vi "cXB_trt-2-dist.vi"(8 "err in":errorcluster, 11 "cXB (e)":T1) -> (0 "errout":errorcluster caption="err out", 3 "cXB (s)":T1)   [LabVIEW 2010]
doc: "Calcul des caractéristiques de la distribution expérimentale : nic (effectifs cumulés), Densité de probabilité f(X), Fonction de répartition F(X) à partir des informations en entrée (n obs. ou nc classes), de l'effectif total (n), et du tableau 1D des effectifs associés (ni) à chaque valeur ou chaque classe."
uses:
  lv_04/commandes/cX.ctl
  lv_04/commandes/cSTA_varid.ctl
  lv_04/commandes/c_TDMS_ch_variable.ctl
  lv_04/commandes/c_TDMS_ch_donnees.ctl
  lv_04/commandes/c0-var-n.ctl
  lv_04/commandes/cSTA_num_do_cr.ctl
  lv_04/commandes/c02-do-num.ctl
  lv_04/commandes/c04-stat-num.ctl
  lv_04/commandes/cSTA_txt_do_cr.ctl
  lv_04/commandes/c02-do-txt.ctl
  lv_04/commandes/c04-stat-txt.ctl
  lv_04/commandes/cSTA_dist.ctl
  lv_04/commandes/c03-dist-S.ctl
  lv_04/commandes/c0-dist-xy.ctl
  lv_04/commandes/c03-dist-T.ctl
  lv_04/commandes/c03-dist-SPC.ctl
  lv_01/lv_01.lvlib
  lv_04/lv_04.lvlib
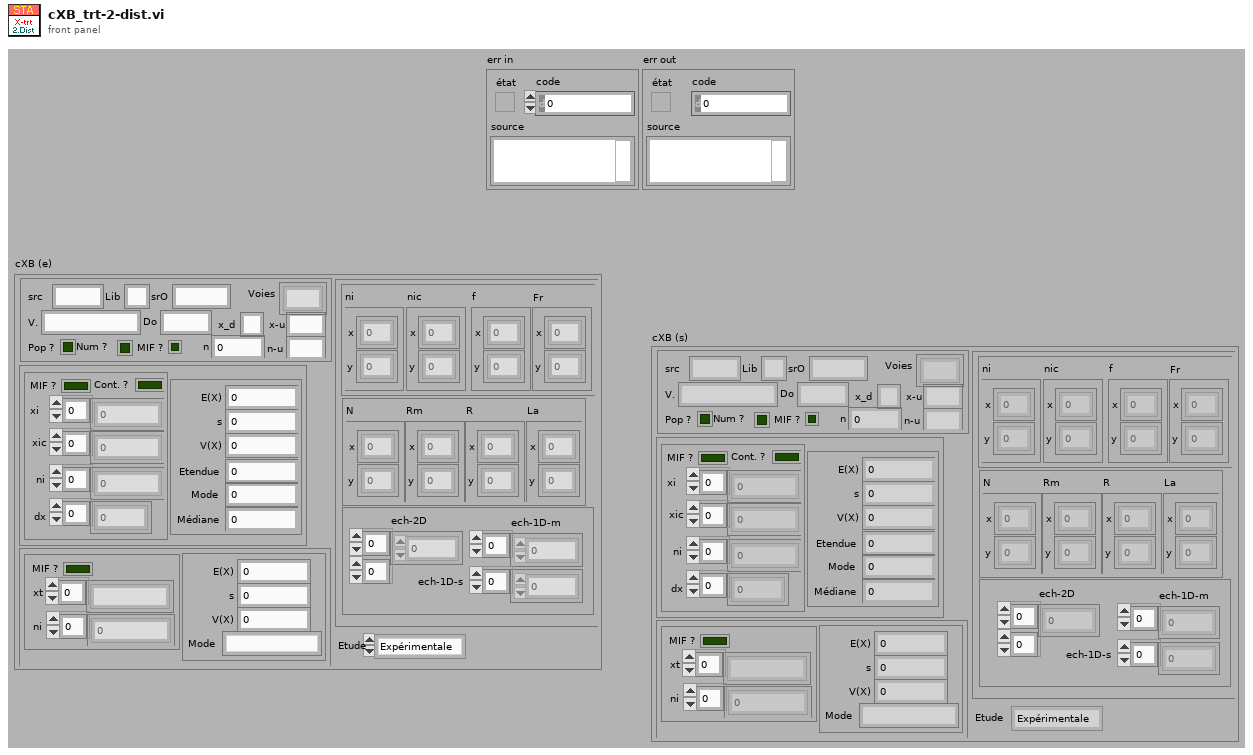
[diagram p1: front panel]
types:
  T1 = typedef "lv_04.lvlib/cX.ctl" = cluster{"src":T2, "num":T6, "txt":T9, "dist":T12, "Etude":enum16{"Expérimentale", "Modèle"}}
  T2 = typedef "lv_04.lvlib/cSTA_varid.ctl" = cluster{"src":string, "Lib":string, "srO":string, "V.":T3, "Voies":string[], "Do":T4, "n":T5, "Num ?":bool, "Pop ?":bool, "x_d":string, "x-u":string, "n-u":string, "MIF ?":bool}
  T3 = typedef "lv_04.lvlib/c_TDMS_ch_variable.ctl" = string
  T4 = typedef "lv_04.lvlib/c_TDMS_ch_donnees.ctl" = string
  T5 = typedef "lv_04.lvlib/c0-var-n.ctl" = i32
  T6 = typedef "lv_04.lvlib/cSTA_num_do_cr.ctl" = cluster{"do":T7, "sta":T8}
  T7 = typedef "lv_04.lvlib/c02-do-num.ctl" = cluster{"MIF ?":bool, "Cont. ?":bool, "xi":dbl[], "xic":dbl[], "ni":u32[], "dx":dbl[]}
  T8 = typedef "lv_04.lvlib/c04-stat-num.ctl" = cluster{"E(X)":dbl, "s":dbl, "V(X) ":dbl, "Etendue":dbl, "Mode":dbl, "Médiane":dbl}
  T9 = typedef "lv_04.lvlib/cSTA_txt_do_cr.ctl" = cluster{"do":T10, "sta":T11}
  T10 = typedef "lv_04.lvlib/c02-do-txt.ctl" = cluster{"xt":string[], "ni":dbl[], "MIF ?":bool}
  T11 = typedef "lv_04.lvlib/c04-stat-txt.ctl" = cluster{"E(X)":dbl, "s":dbl, "V(X) ":dbl, "Mode":string}
  T12 = typedef "lv_04.lvlib/cSTA_dist.ctl" = cluster{"S":T13, "T":T15, "spc":T16}
  T13 = typedef "lv_04.lvlib/c03-dist-S.ctl" = cluster{"nic":T14, "f":T14, "Fr":T14, "ni":T14}
  T14 = typedef "lv_04.lvlib/c0-dist-xy.ctl" = cluster{"x":dbl[], "y":dbl[]}
  T15 = typedef "lv_04.lvlib/c03-dist-T.ctl" = cluster{"N":T14, "Rm":T14, "R":T14, "La":T14}
  T16 = typedef "lv_04.lvlib/c03-dist-SPC.ctl" = cluster{"ech-2D":dbl[][], "ech-1D-m":dbl[], "ech-1D-s":dbl[]}
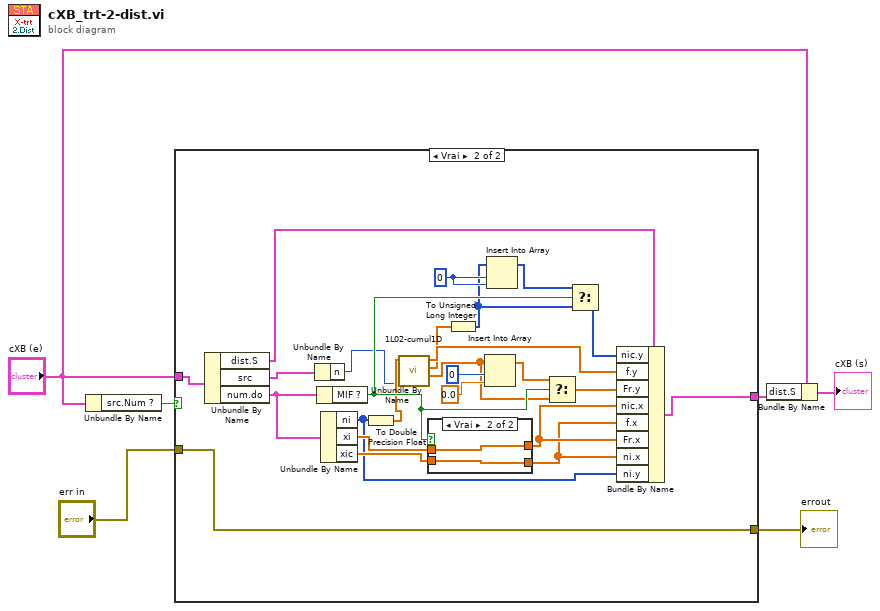
[diagram p0: block diagram]
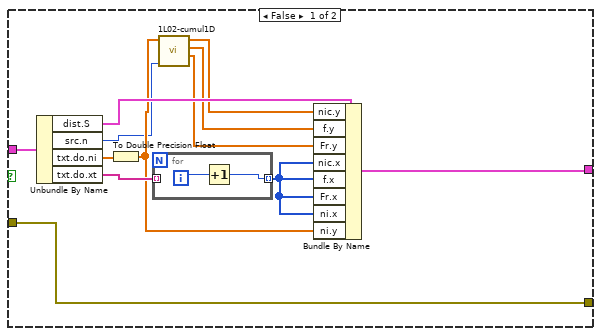
[diagram p2: hidden frame]
diagram:
  n1 = Unbundle By Name("cXB (e)") -> ("src.Num ?"=w6:bool)
  n2 = case shown="Vrai" w6 {
    tunnel: "cXB (e)" -> [w14 w30]
    tunnel: [w13 w28] -> w3
    tunnel: "err in" -> [w12 w27]
    tunnel: [w12 w27] -> w2
    frame False {
      n3 = Unbundle By Name(w14) -> ("dist.S"=w15:T13, "src.n"=w10:T5, "txt.do.ni"=w17:dbl[], "txt.do.xt"=w16:string[])
      n4 = To Double Precision Float(number=w17) -> (double precision float=w11:dbl[])
      n5 = for {
        tunnel: w16 -> [_] mode=indexing
        tunnel: [w19] -> w18 mode=indexing
        i -> [w20]
        n6 = Increment(x=w20) -> (x+1=w19:i32)
      }
      n7 = call "1L02-cumul1D.vi"("som_X"=w10, "X"=w11) -> ("X cum en %"=w7:dbl[], "X en %"=w8:dbl[], "X Cum"=w9:dbl[])  [unwired: 2 in, 1 out]
      n8 = Bundle By Name(cluster=w15, "nic.y"=w9, "f.y"=w8, "Fr.y"=w7, "nic.x"=w18, "f.x"=w18, "Fr.x"=w18, "ni.x"=w18, "ni.y"=w11) -> (w13:T13)
    }
    frame True {
      w34 = 0 ("indice")
      n9 = Unbundle By Name(w30) -> ("dist.S"=w29:T13, "src"=w32:T2, "num.do"=w31:T7)
      n10 = Unbundle By Name(w32) -> ("n"=w25:T5)
      n11 = Unbundle By Name(w31) -> ("MIF ?"=w35:bool)
      n12 = Unbundle By Name(w31) -> ("ni"=w43:u32[], "xi"=w45:dbl[], "xic"=w44:dbl[])
      n13 = To Double Precision Float(number=w43) -> (double precision float=w26:dbl[])
      n14 = call "1L02-cumul1D.vi"("som_X"=w25, "X"=w26) -> ("X cum en %"=w23:dbl[], "X en %"=w21:dbl[], "X Cum"=w24:dbl[])  [unwired: 2 in, 1 out]
      n15 = case shown="Vrai" w35 {
        tunnel: w45 -> [w46 w48]
        tunnel: w44 -> [_ w47]
        tunnel: [w46 w48] -> w38
        tunnel: [w46 w47] -> w37
        frame False {
        }
        frame True {
        }
      }
      n16 = To Unsigned Long Integer(number=w21) -> (unsigned 32bit integer=w22:u32[])
      n17 = Insert Into Array(array=w23, index=0 ("indice"), new element=0.0 ("nouvel élément/sous-tableau")) -> (w40:dbl[])
      n18 = Insert Into Array(array=w22, index=w34, new element=w34) -> (w33:u32[])
      n19 = Select(t=w40, s=w35, f=w23) -> (s? t:f=w39:dbl[])
      n20 = Select(t=w33, s=w35, f=w22) -> (s? t:f=w36:u32[])
      n21 = Bundle By Name(cluster=w29, "nic.y"=w36, "f.y"=w24, "Fr.y"=w39, "nic.x"=w38, "f.x"=w37, "Fr.x"=w38, "ni.x"=w37, "ni.y"=w43) -> (w28:T13)
    }
  }
  "errout" <- w2
  n22 = Bundle By Name(cluster="cXB (e)", "dist.S"=w3) -> (→"cXB (s)":T1)
